vi "Receive.vi"(6 "Timeout":T1={"mode"=enum."Relative", "deadline (ms)"=30000}, 8 "error in (no error)":errorcluster, 9 "request id":u32, 10 "session in":refnum<class "Session.lvclass">, 11 "NI_SFTP.lvlib:posix-rename_openssh.com.lvclass":refnum<class "posix-rename_openssh.com.lvclass">) -> (0 "error out":errorcluster, 1 "unused":i32, 2 "session out":refnum<class "Session.lvclass">, 3 "NI_SFTP.lvlib:posix-rename_openssh.com.lvclass 2":refnum<class "posix-rename_openssh.com.lvclass">)   [LabVIEW 2020, in "NI_SFTP.lvlib" / "posix-rename_openssh.com.lvclass"]
uses:
  <vilib>/net/SFTP/API/Support/Command/posix-rename_openssh.com/posix-rename_openssh.com.lvclass
  <vilib>/net/SFTP/Session/Session.lvclass
  <vilib>/Utility/Deadline/Deadline.ctl
  <vilib>/Utility/Deadline/Mode.ctl
  <vilib>/net/SFTP/API/Support/Command/SSH_FXP_EXTENDED/SSH_FXP_EXTENDED.lvclass
  <vilib>/Utility/Deadline/NI_Deadline.lvlib
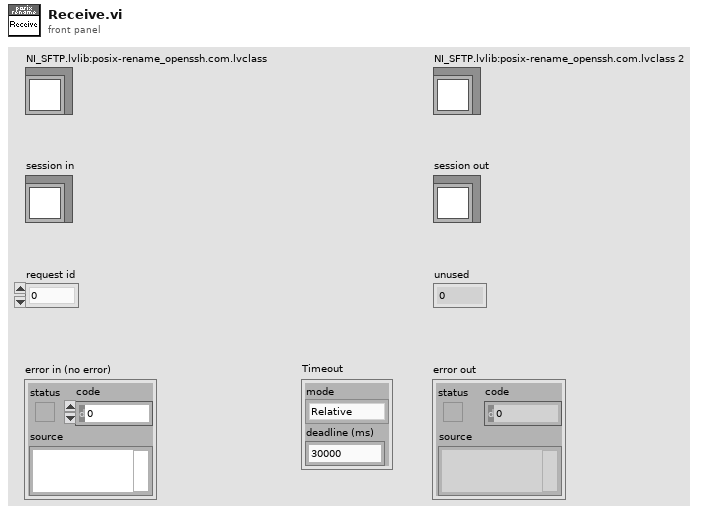
[diagram p1: front panel]
types:
  T1 = typedef "NI_Deadline.lvlib/Deadline.ctl" = cluster{"mode":T2, "deadline (ms)":u32}
  T2 = typedef "NI_Deadline.lvlib/Mode.ctl" = enum16{"Relative", "Use deadline", "Wait forever", "Nonblocking", "N/A"}
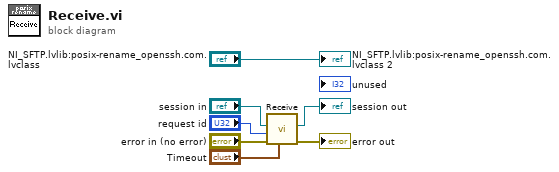
[diagram p0: block diagram]
diagram:
  n1 = call <vilib>:"Receive.vi"("deadline"="Timeout", "error in (no error)"="error in (no error)", "request id"="request id", "session in"="session in") -> ("error out"=→"error out":errorcluster, "session out"=→"session out":refnum<class "Session.lvclass">)  [unwired: 4 in, 2 out]
  "NI_SFTP.lvlib:posix-rename_openssh.com.lvclass 2" <- "NI_SFTP.lvlib:posix-rename_openssh.com.lvclass"
